vi "Teleop.vi"(10 "Match Info":T2={"Autonomous Elapsed Seconds"=0.0, "TeleOp Elapsed Seconds"=0.0, "Disabled Elapsed Seconds"=0.0, "Visited Autonomous"=FALSE, "Visited TeleOp"=FALSE, "Visited Disabled"=FALSE, "Autonomous Settings"={"Autonomous Style"=enum."Independent", "VI Refnum"=refnum}}, 11 "Call Context":T3) -> ()   [LabVIEW 2017]
doc: "This VI is called for each TeleOp packet received from the DS where the robot is not disabled. It is often used to read from the joysticks and update I/O or to update setpoints for timed control loops. It should complete and return within 20 milliseconds or it may miss DS packets."
uses:
  <vilib>/Rock Robotics/WPI/DriverStation/WPI_DriverStationDerivedRobotMode.ctl
  <vilib>/Rock Robotics/WPI/DriverStation/WPI_DriverStationMatch Info.ctl
  TypeDef/ENUM_Arm_Select.ctl
  _SHARE ALL/TypeDef Share All/ENUM_Joystick_Axes.ctl
  _SHARE ALL/TypeDef Share All/CLUSTER_TalonInput.ctl
  System Drivers/Phoenix-LabVIEW/Motor Controller/Controls/CTRE_Phoenix_MotorControl_ControlMode.ctl
  TypeDef/CLUSTER_PID.ctl
  _SHARE ALL/RoboRio Share All/Systems Share All/Joystick/Global_Joystick Write_Data.vi
  Systems/Arm/Global_SM Write_Data Out.vi
  Systems/Lift/Global_SM Write_Data Out.vi
  Systems/Claw Rotation/Global_SM Write_Data Out.vi
  _SHARE ALL/RoboRio Share All/Systems Share All/Joystick/Joystick.lvlib
  Globals/Global_CMD_Drive.vi
  Globals/Global_CMD_Gear.vi
  TypeDef/ENUM_WC_Drive_DriveMode.ctl
  Systems/Lift/Lift.lvlib
  Systems/Claw Rotation/Claw_Rotation.lvlib
  Systems/Arm/Arm.lvlib
panel:
  in  "Zero Encoder":bool
  in  "Arm Control":T1
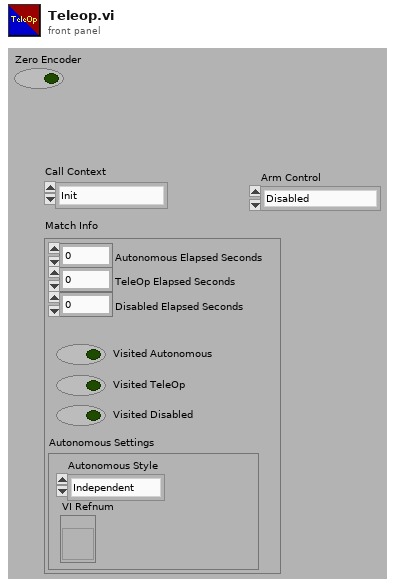
[diagram p1: front panel]
types:
  T1 = typedef "ENUM_Arm_Select.ctl" = enum16{"Disabled", "Arm", "Lift", "Claw Rotation"}
  T2 = typedef "WPI_DriverStationMatch Info.ctl" = cluster{"Autonomous Elapsed Seconds":dbl, "TeleOp Elapsed Seconds":dbl, "Disabled Elapsed Seconds":dbl, "Visited Autonomous":bool, "Visited TeleOp":bool, "Visited Disabled":bool, "Autonomous Settings":cluster{"Autonomous Style":enum16{"Iterative", "Independent"}, "VI Refnum":refnum<vi>}}
  T3 = typedef "WPI_DriverStationDerivedRobotMode.ctl" = enum16{"Init", "Execute", "Stop"}
  T4 = typedef "ENUM_Joystick_Axes.ctl" = enum16{"Left X", "Left Y", "Left Trigger", "Right Trigger", "Right X", "Right Y"}
  T5 = typedef "ENUM_WC_Drive_DriveMode.ctl" = enum16{"Motion Profile", "CrossLineAuto", "VBus", "Stop"}
  T6 = typedef "CLUSTER_CMD_WC_Drive.ctl" = cluster{"Drive_Mode":T5, "VBus":T7, "Profile":T9}
  T7 = typedef "CLUSTER_Drive_ACT Loop_VBus Data.ctl" = cluster{"Drive":T8, "Turbo":bool}
  T8 = typedef "CLUSTER_X and Y.ctl" = cluster{"Steer":dbl, "Throtle":dbl}
  T9 = typedef "CLUSTER_Drive_ACT Loop_Profile Data.ctl" = cluster{"Start":bool}
  T10 = typedef "CLUSTER_TalonInput.ctl" = cluster{"Talon Mode":T11, "Talon Output":dbl, "Zero Encoder":bool, "PID":T12}
  T11 = typedef "CTRE_Phoenix_MotorControl_ControlMode.ctl" = u16
  T12 = typedef "CLUSTER_PID.ctl" = cluster{"P":dbl, "I":dbl, "D":dbl, "F":dbl, "I Zone":dbl}
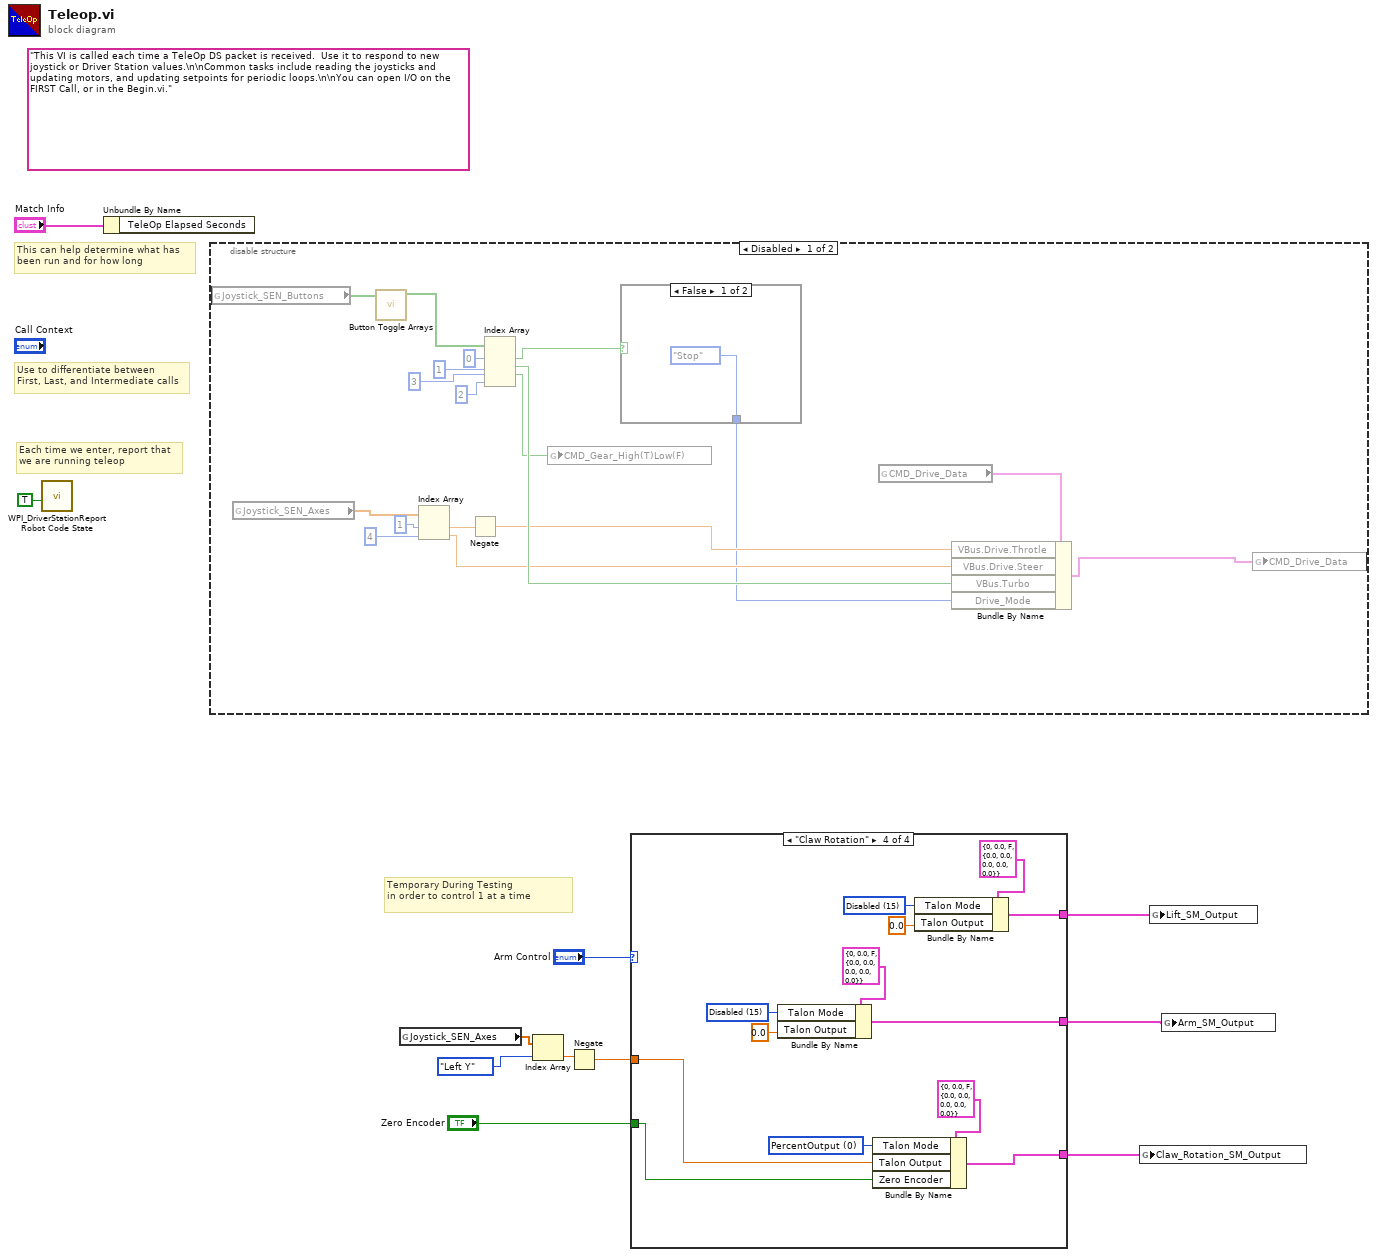
[diagram p0: block diagram]
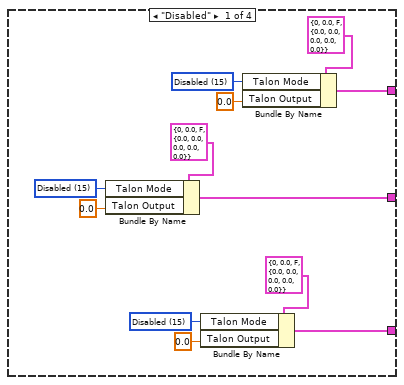
[diagram p2: hidden frame]
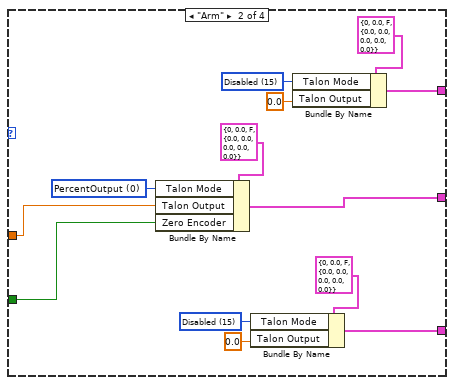
[diagram p3: hidden frame]
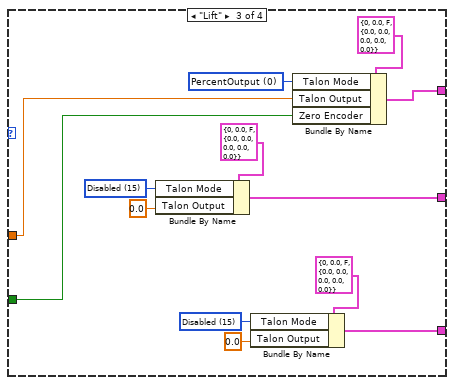
[diagram p4: hidden frame]
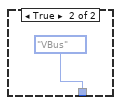
[diagram p5: hidden frame]
diagram:
  (unwired) "This VI is called each time a TeleOp DS packet is received.  Use it to respond to new joystick or Driver Station values.\n\nCommon tasks include reading the joysticks and updating motors, and updating setpoints for periodic loops.\n\nYou can open I/O on the FIRST Call, or in the Begin.vi."
  # "Temporary During Testing\nin order to control 1 at a time"
  # "Each time we enter, report that\nwe are running teleop"
  # "Use to differentiate between\nFirst, Last, and Intermediate calls"
  # "This can help determine what has\nbeen run and for how long"
  n1 = call <vilib>:"WPI_DriverStationReport Robot Code State.vi"("TeleOp"=TRUE ("Autonomous")) -> ()  [unwired: 10 in, 1 out]
  n2 = Unbundle By Name("Match Info") -> ()  [unwired: 1 out]
  n3 = disable-structure shown="Disabled" {
    frame Disabled {
      n4 = global read "Global_Joystick Write_Data.vi" "Joystick_SEN_Buttons"() -> (w17:bool[])
      n5 = global read "Global_Joystick Write_Data.vi" "Joystick_SEN_Axes"() -> (w27:dbl[])
      n6 = call "Button Toggle Arrays.vi"("Joystick_SEN_Buttons"=w17) -> ("Toggle Outputs Out"=w16:bool[])  [unwired: 8 in, 2 out]
      n7 = Index Array(array=w27, index #1=1 ("index"), index #2=4 ("index")) -> (element #1=w21:dbl, element #2=w23:dbl)
      n8 = Negate(x=w21) -> (-x=w20:dbl)
      n9 = Index Array(array=w16, index #1=0 ("index"), index #2=1 ("index"), index #3=3 ("index"), index #4=2 ("index")) -> (element #1=w29:bool, element #2=w25:bool, element #3=w14:bool)  [unwired: 1 out]
      n10 = global write "Global_CMD_Gear.vi" "CMD_Gear_High(T)Low(F)"(w14) -> ()
      n11 = case shown="False" w29 {
        tunnel: [ENUM_WC_Drive_DriveMode."Stop" ("Drive_Mode") ENUM_WC_Drive_DriveMode."VBus" ("Drive_Mode")] -> w12
        frame False {
        }
        frame True {
        }
      }
      n12 = global read "Global_CMD_Drive.vi" "CMD_Drive_Data"() -> (w19:T6)
      n13 = Bundle By Name(cluster=w19, "VBus.Drive.Throtle"=w20, "VBus.Drive.Steer"=w23, "VBus.Turbo"=w25, "Drive_Mode"=w12) -> (w18:T6)
      n14 = global write "Global_CMD_Drive.vi" "CMD_Drive_Data"(w18) -> ()
    }
    frame Enabled {
    }
  }
  n15 = global read "Global_Joystick Write_Data.vi" "Joystick_SEN_Axes"() -> (w5:dbl[])
  n16 = Index Array(array=w5, index=ENUM_Joystick_Axes."Left Y" ("Joystick_Axes")) -> (element=w3:dbl)
  n17 = Negate(x=w3) -> (-x=w2:dbl)
  n18 = case shown="\"Claw Rotation\"" "Arm Control" {
    tunnel: [w34 w49 w61 w74] -> w8
    tunnel: [w33 w48 w60 w73] -> w7
    tunnel: [w32 w47 w59 w72] -> w6
    tunnel: w2 -> [_ w45 w58 w71]
    tunnel: "Zero Encoder" -> [_ w44 w57 w70]
    frame "Disabled" {
      w38 = T11 15 items=["PercentOutput"=0, "Position"=1, "Velocity"=2, "Current"=3, "Follower"=5, "MotionProfile"=6, "MotionMagic"=7, "MotionMagicArc"=8, "MotionProfileArc"=10, "Disabled"=15] ("Talon Mode")
      w39 = T11 15 items=["PercentOutput"=0, "Position"=1, "Velocity"=2, "Current"=3, "Follower"=5, "MotionProfile"=6, "MotionMagic"=7, "MotionMagicArc"=8, "MotionProfileArc"=10, "Disabled"=15] ("Talon Mode")
      w42 = T11 15 items=["PercentOutput"=0, "Position"=1, "Velocity"=2, "Current"=3, "Follower"=5, "MotionProfile"=6, "MotionMagic"=7, "MotionMagicArc"=8, "MotionProfileArc"=10, "Disabled"=15] ("Talon Mode")
      n19 = Bundle By Name(cluster=T10 {"Talon Mode"=0, "Talon Output"=0.0, "Zero Encoder"=FALSE, "PID"={"P"=0.0, "I"=0.0, "D"=0.0, "F"=0.0, "I Zone"=0.0}} ("Lift_SM_Output"), "Talon Mode"=w39, "Talon Output"=0.0) -> (w32:T10)
      n20 = Bundle By Name(cluster=T10 {"Talon Mode"=0, "Talon Output"=0.0, "Zero Encoder"=FALSE, "PID"={"P"=0.0, "I"=0.0, "D"=0.0, "F"=0.0, "I Zone"=0.0}} ("Lift_SM_Output"), "Talon Mode"=w38, "Talon Output"=0.0) -> (w34:T10)
      n21 = Bundle By Name(cluster=T10 {"Talon Mode"=0, "Talon Output"=0.0, "Zero Encoder"=FALSE, "PID"={"P"=0.0, "I"=0.0, "D"=0.0, "F"=0.0, "I Zone"=0.0}} ("Lift_SM_Output"), "Talon Mode"=w42, "Talon Output"=0.0) -> (w33:T10)
    }
    frame "Arm" {
      w46 = T11 0 items=["PercentOutput"=0, "Position"=1, "Velocity"=2, "Current"=3, "Follower"=5, "MotionProfile"=6, "MotionMagic"=7, "MotionMagicArc"=8, "MotionProfileArc"=10, "Disabled"=15] ("Talon Mode")
      w53 = T11 15 items=["PercentOutput"=0, "Position"=1, "Velocity"=2, "Current"=3, "Follower"=5, "MotionProfile"=6, "MotionMagic"=7, "MotionMagicArc"=8, "MotionProfileArc"=10, "Disabled"=15] ("Talon Mode")
      w55 = T11 15 items=["PercentOutput"=0, "Position"=1, "Velocity"=2, "Current"=3, "Follower"=5, "MotionProfile"=6, "MotionMagic"=7, "MotionMagicArc"=8, "MotionProfileArc"=10, "Disabled"=15] ("Talon Mode")
      n22 = Bundle By Name(cluster=T10 {"Talon Mode"=0, "Talon Output"=0.0, "Zero Encoder"=FALSE, "PID"={"P"=0.0, "I"=0.0, "D"=0.0, "F"=0.0, "I Zone"=0.0}} ("Lift_SM_Output"), "Talon Mode"=w46, "Talon Output"=w45, "Zero Encoder"=w44) -> (w47:T10)
      n23 = Bundle By Name(cluster=T10 {"Talon Mode"=0, "Talon Output"=0.0, "Zero Encoder"=FALSE, "PID"={"P"=0.0, "I"=0.0, "D"=0.0, "F"=0.0, "I Zone"=0.0}} ("Lift_SM_Output"), "Talon Mode"=w53, "Talon Output"=0.0) -> (w49:T10)
      n24 = Bundle By Name(cluster=T10 {"Talon Mode"=0, "Talon Output"=0.0, "Zero Encoder"=FALSE, "PID"={"P"=0.0, "I"=0.0, "D"=0.0, "F"=0.0, "I Zone"=0.0}} ("Lift_SM_Output"), "Talon Mode"=w55, "Talon Output"=0.0) -> (w48:T10)
    }
    frame "Lift" {
      w65 = T11 15 items=["PercentOutput"=0, "Position"=1, "Velocity"=2, "Current"=3, "Follower"=5, "MotionProfile"=6, "MotionMagic"=7, "MotionMagicArc"=8, "MotionProfileArc"=10, "Disabled"=15] ("Talon Mode")
      w66 = T11 15 items=["PercentOutput"=0, "Position"=1, "Velocity"=2, "Current"=3, "Follower"=5, "MotionProfile"=6, "MotionMagic"=7, "MotionMagicArc"=8, "MotionProfileArc"=10, "Disabled"=15] ("Talon Mode")
      w68 = T11 0 items=["PercentOutput"=0, "Position"=1, "Velocity"=2, "Current"=3, "Follower"=5, "MotionProfile"=6, "MotionMagic"=7, "MotionMagicArc"=8, "MotionProfileArc"=10, "Disabled"=15] ("Talon Mode")
      n25 = Bundle By Name(cluster=T10 {"Talon Mode"=0, "Talon Output"=0.0, "Zero Encoder"=FALSE, "PID"={"P"=0.0, "I"=0.0, "D"=0.0, "F"=0.0, "I Zone"=0.0}} ("Lift_SM_Output"), "Talon Mode"=w66, "Talon Output"=0.0) -> (w59:T10)
      n26 = Bundle By Name(cluster=T10 {"Talon Mode"=0, "Talon Output"=0.0, "Zero Encoder"=FALSE, "PID"={"P"=0.0, "I"=0.0, "D"=0.0, "F"=0.0, "I Zone"=0.0}} ("Lift_SM_Output"), "Talon Mode"=w65, "Talon Output"=0.0) -> (w61:T10)
      n27 = Bundle By Name(cluster=T10 {"Talon Mode"=0, "Talon Output"=0.0, "Zero Encoder"=FALSE, "PID"={"P"=0.0, "I"=0.0, "D"=0.0, "F"=0.0, "I Zone"=0.0}} ("Lift_SM_Output"), "Talon Mode"=w68, "Talon Output"=w58, "Zero Encoder"=w57) -> (w60:T10)
    }
    frame "Claw Rotation" {
      w77 = T11 0 items=["PercentOutput"=0, "Position"=1, "Velocity"=2, "Current"=3, "Follower"=5, "MotionProfile"=6, "MotionMagic"=7, "MotionMagicArc"=8, "MotionProfileArc"=10, "Disabled"=15] ("Talon Mode")
      w78 = T11 15 items=["PercentOutput"=0, "Position"=1, "Velocity"=2, "Current"=3, "Follower"=5, "MotionProfile"=6, "MotionMagic"=7, "MotionMagicArc"=8, "MotionProfileArc"=10, "Disabled"=15] ("Talon Mode")
      w81 = T11 15 items=["PercentOutput"=0, "Position"=1, "Velocity"=2, "Current"=3, "Follower"=5, "MotionProfile"=6, "MotionMagic"=7, "MotionMagicArc"=8, "MotionProfileArc"=10, "Disabled"=15] ("Talon Mode")
      n28 = Bundle By Name(cluster=T10 {"Talon Mode"=0, "Talon Output"=0.0, "Zero Encoder"=FALSE, "PID"={"P"=0.0, "I"=0.0, "D"=0.0, "F"=0.0, "I Zone"=0.0}} ("Lift_SM_Output"), "Talon Mode"=w78, "Talon Output"=0.0) -> (w72:T10)
      n29 = Bundle By Name(cluster=T10 {"Talon Mode"=0, "Talon Output"=0.0, "Zero Encoder"=FALSE, "PID"={"P"=0.0, "I"=0.0, "D"=0.0, "F"=0.0, "I Zone"=0.0}} ("Lift_SM_Output"), "Talon Mode"=w77, "Talon Output"=w71, "Zero Encoder"=w70) -> (w74:T10)
      n30 = Bundle By Name(cluster=T10 {"Talon Mode"=0, "Talon Output"=0.0, "Zero Encoder"=FALSE, "PID"={"P"=0.0, "I"=0.0, "D"=0.0, "F"=0.0, "I Zone"=0.0}} ("Lift_SM_Output"), "Talon Mode"=w81, "Talon Output"=0.0) -> (w73:T10)
    }
  }
  n31 = global write "Global_SM Write_Data Out.vi" "Claw_Rotation_SM_Output"(w8) -> ()
  n32 = global write "Global_SM Write_Data Out.vi" "Lift_SM_Output"(w7) -> ()
  n33 = global write "Global_SM Write_Data Out.vi" "Arm_SM_Output"(w6) -> ()
